vi "IndexControl.vi"(8 "Power":dbl, 10 "Backward":bool, 11 "Forward":bool) -> (2 "Numeric":dbl)   [LabVIEW 2011]
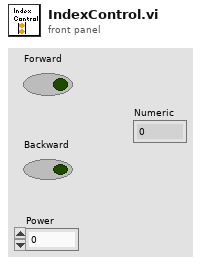
[diagram p1: front panel]
types:
  T1 = typedef "WPI_DigitalInputDevRef.ctl" = cluster{"DevStatus":errorcluster, "DIO Channel":T2, "Digital Module":T3}
  T2 = typedef "FPGA_DIOChannel.ctl" = enum8{"DIO 1", "DIO 2", "DIO 3", "DIO 4", "DIO 5", "DIO 6", "DIO 7", "DIO 8", "DIO 9", "DIO 10", "DIO 11", "DIO 12", "DIO 13", "DIO 14", "Invalid"}
  T3 = typedef "FPGA_TypedefDigitalModule.ctl" = enum16{"Digital Module 1", "Digital Module 2"}
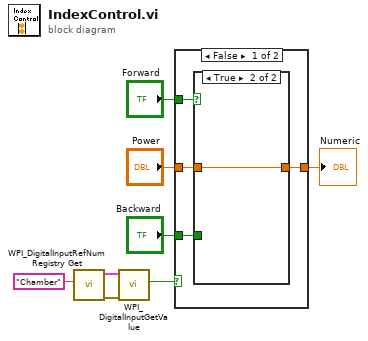
[diagram p0: block diagram]
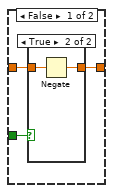
[diagram p2: hidden frame]
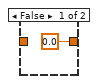
[diagram p3: hidden frame]
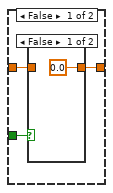
[diagram p5: hidden frame]
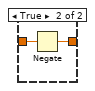
[diagram p6: hidden frame]
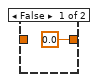
[diagram p7: hidden frame]
diagram:
  n1 = call <vilib>:"WPI_DigitalInputRefNum Registry Get.vi"("refnum name"="Chamber") -> ("error out"=w4:errorcluster, "DigitalInputDevRef"=w3:T1)  [unwired: 9 in]
  n2 = call <vilib>:"WPI_DigitalInputGetValue.vi"("error in (no error)"=w4, "DigitalInputDevRef"=w3) -> ("Value"=w2:bool)  [unwired: 7 in, 2 out]
  n3 = case shown="False" w2 {
    tunnel: "Forward" -> [w12 w21]
    tunnel: "Power" -> [w11 w22]
    tunnel: [w10 w23] -> w6
    tunnel: "Backward" -> [w9 w20]
    frame False {
      n4 = case shown="True" w12 {
        tunnel: w11 -> [w14 w19]
        tunnel: [w13 w19] -> w10
        tunnel: w9 -> [w15 _]
        frame False {
          n5 = case shown="True" w15 {
            tunnel: w14 -> [_ w18]
            tunnel: [0.0 w17] -> w13
            frame False {
            }
            frame True {
              n6 = Negate(x=w18) -> (-x=w17:dbl)
            }
          }
        }
        frame True {
        }
      }
    }
    frame True {
      n7 = case shown="True" w21 {
        tunnel: w22 -> [w26 w30]
        tunnel: [w25 w32] -> w23
        tunnel: w20 -> [w24 w31]
        frame False {
          n8 = case shown="False" w24 {
            tunnel: w26 -> [_ w29]
            tunnel: [0.0 w28] -> w25
            frame False {
            }
            frame True {
              n9 = Negate(x=w29) -> (-x=w28:dbl)
            }
          }
        }
        frame True {
          n10 = case shown="True" w31 {
            tunnel: [0.0 w34] -> w32
            tunnel: w30 -> [_ w34]
            frame False {
            }
            frame True {
            }
          }
        }
      }
    }
  }
  "Numeric" <- w6
